vi "Get TPCANHandle.vi"(11 "PCAN Basic Base Configure Strategy in":refnum<class "PCAN Basic Base Configure Strategy.lvclass">) -> (2 "TPCANHandle":T1=81 items=["PCAN_NONEBUS"=0, "PCAN_USBBUS1"=81, "PCAN_USBBUS2"=82, "PCAN_USBBUS3"=83, "PCAN_USBBUS4"=84, "PCAN_USBBUS5"=85, "PCAN_USBBUS6"=86, "PCAN_USBBUS7"=87, "PCAN_USBBUS8"=88, "PCAN_USBBUS9"=1289, "PCAN_USBBUS10"=1290, "PCAN_USBBUS11"=1291, "PCAN_USBBUS12"=1292, "PCAN_USBBUS13"=1293, "PCAN_USBBUS14"=1294, "PCAN_USBBUS15"=1295, "PCAN_USBBUS16"=1296], 3 "PCAN Basic Base Configure Strategy out":refnum<class "PCAN Basic Base Configure Strategy.lvclass">)   [LabVIEW 2025, in "PCAN Basic Base Configure Strategy.lvclass"]
uses:
  PCAN Basic Base Configure Strategy.lvclass
  <instrlib>/Peter/PCAN Basic/TPCANHandle.ctl
  PCAN Basic Base Configure Strategy.lvclass/PCAN Basic Base Configure Strategy.ctl
  <instrlib>/Peter/PCAN Basic/PCANBasic.lvlib
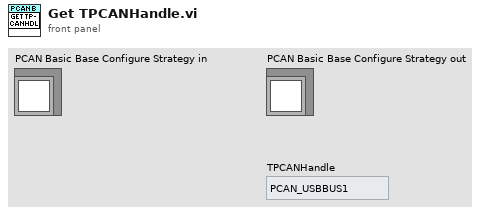
[diagram p1: front panel]
types:
  T1 = typedef "PCANBasic.lvlib/TPCANHandle.ctl" = u16
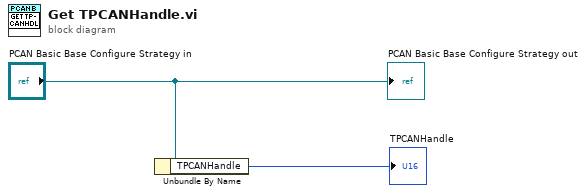
[diagram p0: block diagram]
diagram:
  n1 = Unbundle By Name("PCAN Basic Base Configure Strategy in") -> ("TPCANHandle"=→"TPCANHandle":T1)
  "PCAN Basic Base Configure Strategy out" <- "PCAN Basic Base Configure Strategy in"
